vi "Update Device Properties Table.vi"(0 "session in":refnum<k21>, 5 "device":refnum<k21>, 7 "device properties":refnum<vi>, 11 "error in (no error)":errorcluster) -> (4 "session out":refnum<k21>, 15 "error out":errorcluster)   [LabVIEW 2017]
uses:
  <vilib>/Utility/error.llb/DialogType.ctl
  <resource>/objmgr/slsc.rc
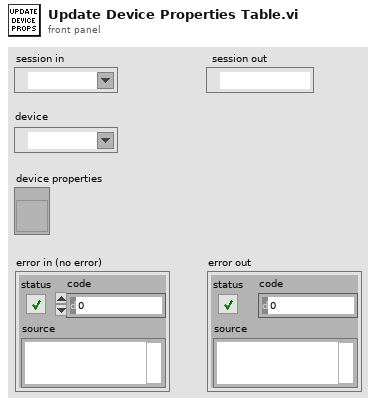
[diagram p1: front panel]
types:
  T1 = typedef "DialogType.ctl" = u16
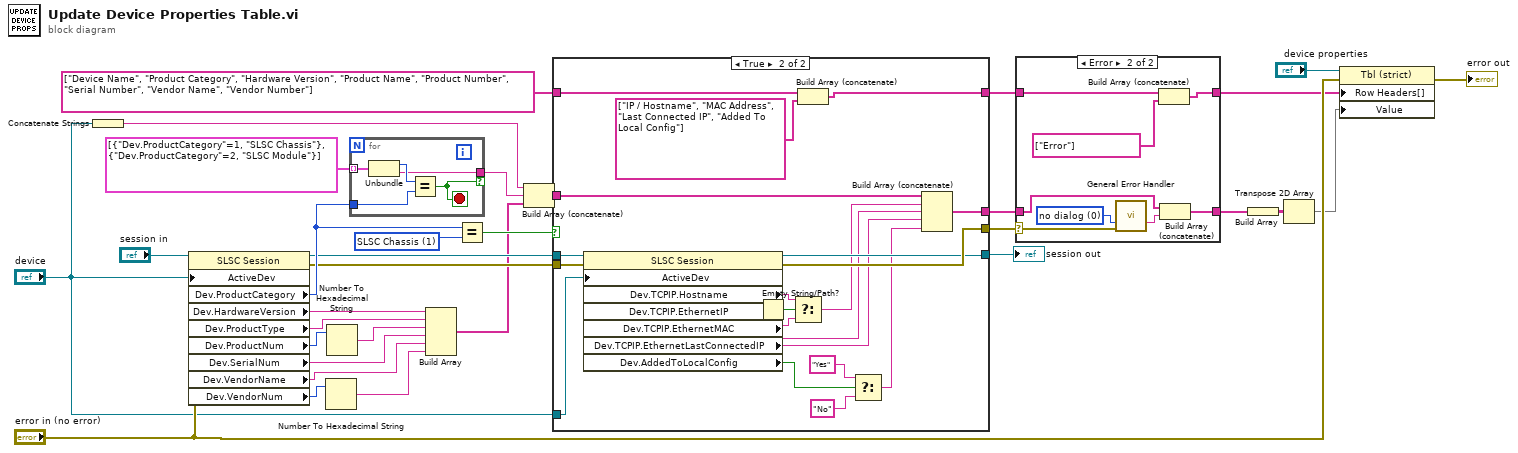
[diagram p0: block diagram]
diagram:
  w24 = 1 items=["Unknown", "SLSC Chassis", "SLSC Module"] ("Dev.ProductCategory")
  n1 = Concatenate Strings("device") -> (w2:string)
  n2 = property class="SLSC Session"(reference="session in", error in="error in (no error)", "ActiveDev"="device") -> (reference out=w21:refnum<k21>, error out=w20:errorcluster, "Dev.ProductCategory"=w23:i32, "Dev.HardwareVersion"=w1:string, "Dev.ProductType"=w29:string, "Dev.ProductNum"=w32:u32, "Dev.SerialNum"=w27:string, "Dev.VendorName"=w26:string, "Dev.VendorNum"=w31:u32)
  n3 = Number To Hexadecimal String(2:w31) -> (0:w25:string)  [unwired: 1 in]
  n4 = Number To Hexadecimal String(2:w32) -> (0:w28:string)  [unwired: 1 in]
  n5 = for {
    tunnel: w23 -> [w37]
    tunnel: cluster{"Dev.ProductCategory":i32, string}[] [{"Dev.ProductCategory"=1, "SLSC Chassis"}, {"Dev.ProductCategory"=2, "SLSC Module"}] -> [w36] mode=indexing
    tunnel: [w34] -> w5 if=w33
    stop <- w33 stop-if-true
    n6 = Unbundle(w36) -> ("Dev.ProductCategory"=w35:i32, w34:string)
    n7 = Equal?(x=w35, y=w37) -> (x = y?=w33:bool)
  }
  n8 = Build Array(w1, w29, w28, w27, w26, w25) -> (w4:string[])
  n9 = Equal?(x=w23, y=w24) -> (x = y?=w22:bool)
  n10 = Build Array (concatenate)(w2, w5, w4) -> (w3:string[])
  n11 = case shown="True" w22 {
    tunnel: w21 -> [w41 w61]
    tunnel: w20 -> [w40 w60]
    tunnel: [w40 w59] -> w19
    tunnel: [w41 w58] -> w14
    tunnel: "device" -> [_ w52]
    tunnel: string[] ["Device Name", "Product Category", "Hardware Version", "Product Name", "Product Number", "Serial Number", "Vendor Name", "Vendor Number"] -> [w39 w51]
    tunnel: [w39 w49] -> w11
    tunnel: w3 -> [w38 w48]
    tunnel: [w38 w47] -> w9
    frame False {
    }
    frame True {
      n12 = property class="SLSC Session"(reference=w61, error in=w60, "ActiveDev"=w52) -> (reference out=w58:refnum<k21>, error out=w59:errorcluster, "Dev.TCPIP.Hostname"=w56:string, "Dev.TCPIP.EthernetIP"=w55:string, "Dev.TCPIP.EthernetMAC"=w53:string, "Dev.TCPIP.EthernetLastConnectedIP"=w46:string, "Dev.AddedToLocalConfig"=w45:bool)
      n13 = Empty String/Path?(string/path=w55) -> (empty?=w57:bool)
      n14 = Select(t=w56, s=w57, f=w55) -> (s? t:f=w54:string)
      n15 = Build Array (concatenate)(w51, string[] ["IP / Hostname", "MAC Address", "Last Connected IP", "Added To Local Config"]) -> (w49:string[])
      n16 = Select(t="Yes" ("Dev.TCPIP.EthernetLastConnectedIP"), s=w45, f="No" ("Dev.TCPIP.EthernetLastConnectedIP")) -> (s? t:f=w42:string)
      n17 = Build Array (concatenate)(w48, w54, w53, w46, w42) -> (w47:string[])
    }
  }
  "session out" <- w14
  n18 = case shown="Error" w19 {
    selector: w19 -> [_ w70]
    tunnel: w11 -> [w63 w68]
    tunnel: [w63 w66] -> w10
    tunnel: w9 -> [w62 w65]
    tunnel: [w62 w64] -> w8
    frame No Error {
    }
    frame Error {
      w71 = T1 0 items=["no dialog", "OK message", "continue or stop message", "OK message + warnings", "continue/stop + warnings"] ("type of dialog (OK msg:1)")
      n19 = call <vilib>:"General Error Handler.vi"("type of dialog (OK msg:1)"=w71, "error in (no error)"=w70) -> ("message"=w69:string)  [unwired: 9 in, 4 out]
      n20 = Build Array (concatenate)(w68, string[] ["Error"]) -> (w66:string[])
      n21 = Build Array (concatenate)(w65, w69) -> (w64:string[])
    }
  }
  n22 = Build Array(w8) -> (w7:string[][])
  n23 = Transpose 2D Array(2D array=w7) -> (transposed array=w6:string[][])
  n24 = property class="Tbl (strict)"(reference="device properties", error in="error in (no error)", "Row Headers[]"=w10, "Value"=w6) -> (error out=→"error out":errorcluster)  [unwired: 1 out]
